vi "VDH-gatherDataForCalibration.vi"(8 "error in (no error)":errorcluster, 10 "VNA data":T1, 11 "VDH-VNA_data_handler in":refnum<class "VDH-VNA_data_handler.lvclass">) -> (0 "error out":errorcluster, 3 "VDH-VNA_data_handler out":refnum<class "VDH-VNA_data_handler.lvclass">)   [LabVIEW 2020, in "VDH-VNA_data_handler.lvlib" / "VDH-VNA_data_handler.lvclass"]
uses:
  VDH-VNA_data_handler.lvclass
  classes/vna-drivers/liteVNA/VD-VNA_data.ctl
  VDH-VNA_data_handler.lvclass/VDH-VNA_data_handler.ctl
  classes/vna-drivers/liteVNA/VD-LV-LiteVNA.lvclass
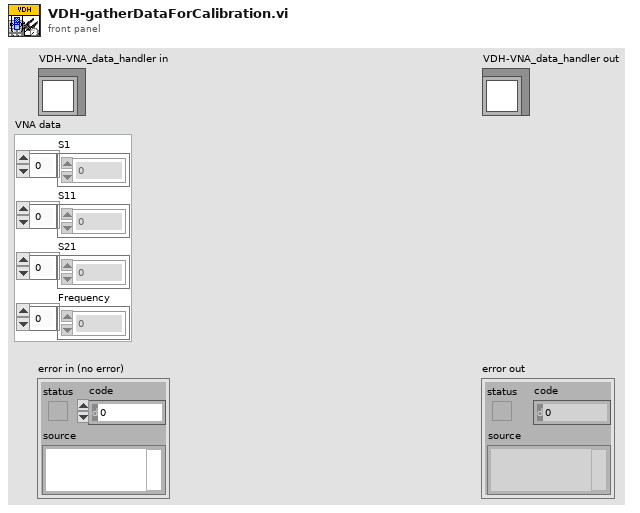
[diagram p1: front panel]
types:
  T1 = typedef "VD-LV-LiteVNA.lvclass/VD-VNA_data.ctl" = cluster{"S1":cdb[], "S11":cdb[], "S21":cdb[], "Frequency":u64[]}
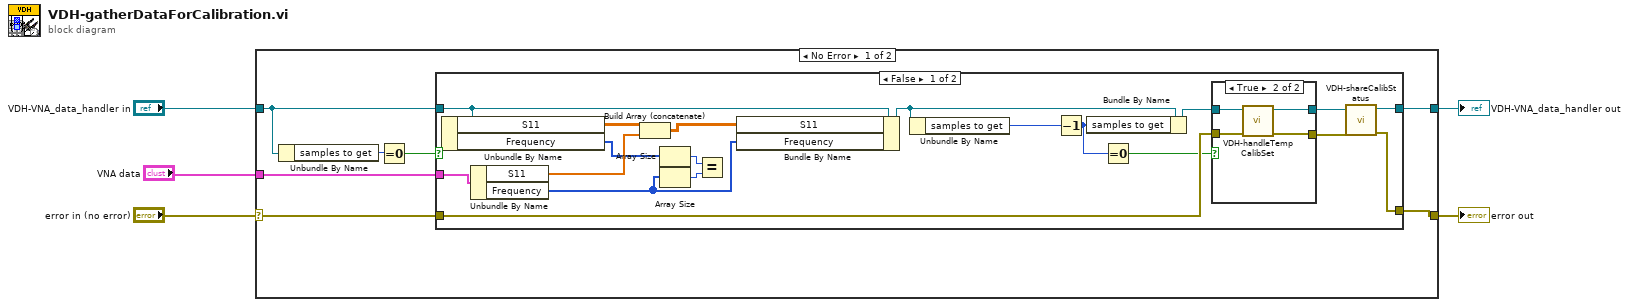
[diagram p0: block diagram]
diagram:
  n1 = case shown="No Error" "error in (no error)" {
    selector: "error in (no error)" -> [w11 w41]
    tunnel: [w9 w41] -> w4
    tunnel: [w10 w40] -> w2
    tunnel: "VDH-VNA_data_handler in" -> [w8 w40]
    tunnel: "VNA data" -> [w12 _]
    frame No Error {
      n2 = Unbundle By Name(w8) -> ("samples to get"=w7:u8)
      n3 = Equal To 0?(x=w7) -> (x = 0?=w6:bool)
      n4 = case shown="False" w6 {
        tunnel: w12 -> [w29 _]
        tunnel: w11 -> [w25 w38]
        tunnel: [w20 w39] -> w10
        tunnel: [w19 w38] -> w9
        tunnel: w8 -> [w17 w39]
        frame False {
          n5 = Unbundle By Name(w17) -> ("S11"=w31:cdb[][], "Frequency"=w16:u64[])
          n6 = Unbundle By Name(w29) -> ("S11"=w28:cdb[], "Frequency"=w15:u64[])
          n7 = Build Array (concatenate)(w31, w28) -> (w30:cdb[][])
          n8 = Array Size(array=w16) -> (size(s)=w14:i32)
          n9 = Array Size(array=w15) -> (size(s)=w13:i32)
          n10 = Equal?(x=w14, y=w13) -> ()  [unwired: 1 out]
          n11 = Bundle By Name(cluster=w17, "S11"=w30, "Frequency"=w15) -> (w27:refnum<class "VDH-VNA_data_handler.lvclass">)
          n12 = Unbundle By Name(w27) -> ("samples to get"=w18:u8)
          n13 = Decrement(x=w18) -> (x-1=w24:u8)
          n14 = Bundle By Name(cluster=w27, "samples to get"=w24) -> (w26:refnum<class "VDH-VNA_data_handler.lvclass">)
          n15 = Equal To 0?(x=w24) -> (x = 0?=w23:bool)
          n16 = case shown="True" w23 {
            tunnel: w26 -> [w33 w37]
            tunnel: [w33 w36] -> w21
            tunnel: w25 -> [w32 w35]
            tunnel: [w32 w34] -> w22
            frame False {
            }
            frame True {
              n17 = call "VDH-handleTempCalibSet.vi"("error in (no error)"=w35, "VDH-VNA_data_handler in"=w37) -> ("error out"=w34:errorcluster, "VDH-VNA_data_handler out"=w36:refnum<class "VDH-VNA_data_handler.lvclass">)  [unwired: 8 in]
            }
          }
          n18 = call "VDH-shareCalibStatus.vi"("error in (no error)"=w22, "VDH-VNA_data_handler in"=w21) -> ("error out"=w19:errorcluster, "VDH-VNA_data_handler out"=w20:refnum<class "VDH-VNA_data_handler.lvclass">)  [unwired: 8 in]
        }
        frame True {
        }
      }
    }
    frame Error {
    }
  }
  "error out" <- w4
  "VDH-VNA_data_handler out" <- w2
